vi "Find Match Values.vi"(6 "Text File String":string[][](array[string]), 7 "Row Index":i32, 9 "New Array Index":i32, 10 "Blank Array":dbl[](array[numeric]), 11 "Pattern Match?":bool) -> (2 "index out":i32, 3 "Array of Values":dbl[](array[numeric]))   [LabVIEW 2020]
uses:
  <vilib>/Analysis/NI_AALBase.lvlib
panel:
  out "Array":dbl[](array[numeric])
  out "Building Array":dbl[](array[numeric])
  out "Column Index":i32
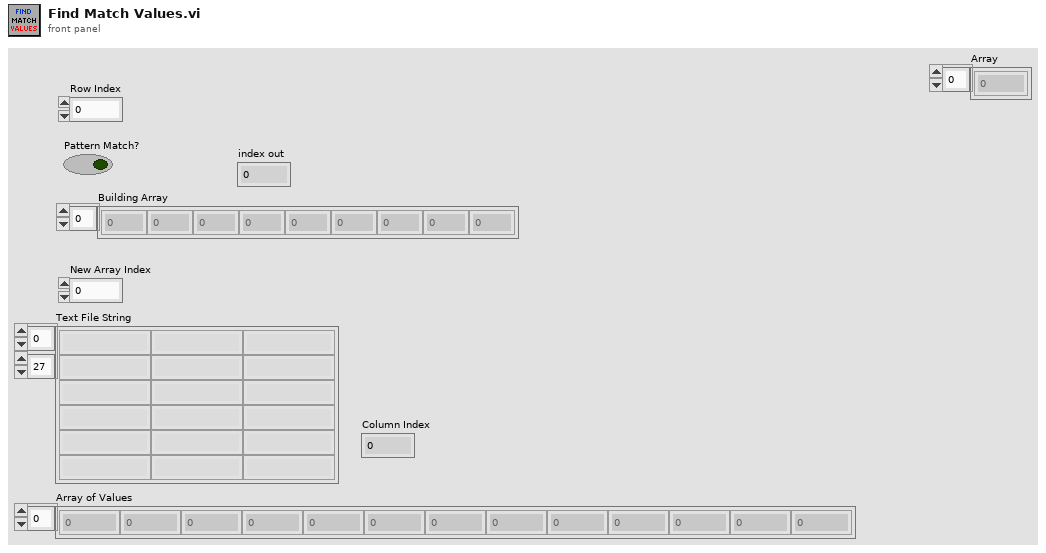
[diagram p1: front panel]
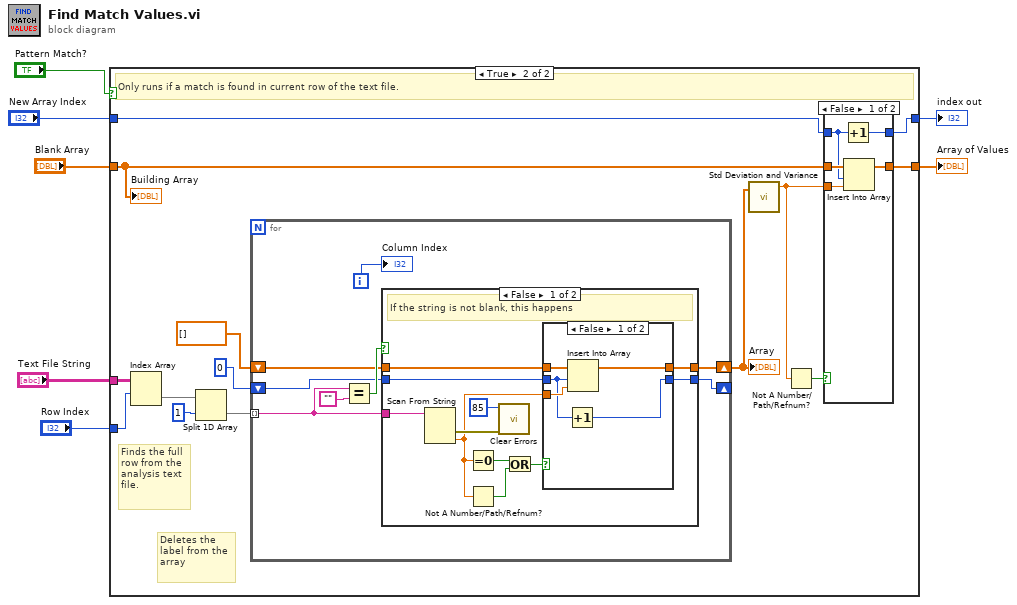
[diagram p0: block diagram]
diagram:
  n1 = case shown="True" "Pattern Match?" {
    tunnel: "Text File String" -> [_ w22]
    tunnel: "Row Index" -> [_ w23]
    tunnel: "Blank Array" -> [w8 w15]
    tunnel: "New Array Index" -> [w9 w14]
    tunnel: [w9 w13] -> w5
    tunnel: [w8 w12] -> w6
    frame False {
      # "If there is no match, nothing happens."
    }
    frame True {
      # "Deletes the label from the array"
      # "Finds the full row from the analysis text file."
      # "Only runs if a match is found in current row of the text file."
      n2 = Index Array(array=w22, index (row)=w23) -> (element=w21:string[])  [unwired: 1 in]
      n3 = Split 1D Array(array=w21, index=1) -> (second subarray=w19:string[])  [unwired: 1 out]
      n4 = for {
        tunnel: w19 -> [w36] mode=indexing
        shift-right: [w35] -> _
        shift-left: 0 ("index") -> [w31]
        shift-right: [w33] -> w16
        shift-left: dbl[] [] ("Array") -> [w34]
        i -> [w32]
        n5 = Equal?(x=w36, y="") -> (x = y?=w37:bool)
        n6 = case shown="False" w37 {
          tunnel: w36 -> [w49 _]
          tunnel: w31 -> [w46 w58]
          tunnel: [w43 w58] -> w35
          tunnel: w34 -> [w48 w57]
          tunnel: [w47 w57] -> w33
          frame False {
            # "If the string is not blank, this happens"
            n7 = Scan From String(input string=w49) -> (error out=w45:errorcluster, output 1=w42:dbl)  [unwired: 4 in, 2 out]
            n8 = Equal To 0?(x=w42) -> (x = 0?=w40:bool)
            n9 = Not A Number/Path/Refnum?(number/path/refnum=w42) -> (NaN/Path/Refnum?=w41:bool)
            n10 = call <vilib>:"Clear Errors.vi"("error in (no error)"=w45, "specific error code to clear (0: all)"=85) -> ()  [unwired: 4 in, 2 out]
            n11 = Or(x=w40, y=w41) -> (x .or. y?=w39:bool)
            n12 = case shown="False" w39 {
              tunnel: w48 -> [w54 w56]
              tunnel: [w53 w56] -> w47
              tunnel: w46 -> [w50 w55]
              tunnel: w42 -> [w52 _]
              tunnel: [w51 w55] -> w43
              frame False {
                n13 = Increment(x=w50) -> (x+1=w51:i32)
                n14 = Insert Into Array "Insert Into Array"(array=w54, index=w50, new element=w52) -> (w53:dbl[])
              }
              frame True {
              }
            }
          }
          frame True {
            # "If the string is blank, nothing happens"
          }
        }
        "Column Index" <- w32
      }
      "Array" <- w16
      n15 = call <vilib>:"Std Deviation and Variance.vi"("X"=w16) -> ("mean"=w11:dbl)  [unwired: 1 in, 2 out]
      n16 = Not A Number/Path/Refnum?(number/path/refnum=w11) -> (NaN/Path/Refnum?=w10:bool)
      n17 = case shown="False" w10 {
        tunnel: w15 -> [w28 w29]
        tunnel: w14 -> [w27 w30]
        tunnel: [w26 w30] -> w13
        tunnel: w11 -> [w25 _]
        tunnel: [w24 w29] -> w12
        frame False {
          n18 = Increment(x=w27) -> (x+1=w26:i32)
          n19 = Insert Into Array(array=w28, index=w27, new element=w25) -> (w24:dbl[])
        }
        frame True {
        }
      }
      "Building Array" <- w15
    }
  }
  "Array of Values" <- w6
  "index out" <- w5
